vi "Popup.vi"(8 "error in (no error)":errorcluster, 10 "MSG":string, 11 "Popup in":refnum<class "Popup.lvclass">) -> (0 "error out":errorcluster, 3 "Popup out":refnum<class "Popup.lvclass">)   [LabVIEW 2020, in "Test-Client.lvlib" / "Popup.lvclass"]
uses:
  Popup.lvclass
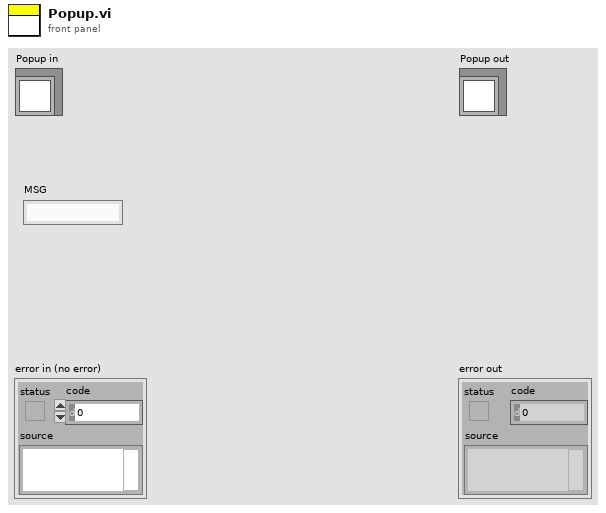
[diagram p1: front panel]
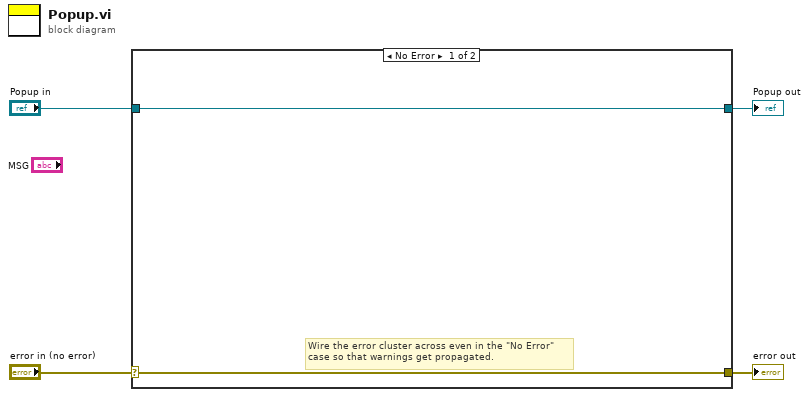
[diagram p0: block diagram]
diagram:
  n1 = case shown="No Error" "error in (no error)" {
    selector: "error in (no error)" -> [w5 w8]
    tunnel: [w5 w8] -> w3
    tunnel: [w6 w7] -> w1
    tunnel: "Popup in" -> [w6 w7]
    frame No Error {
      # "Wire the error cluster across even in the \"No Error\"\ncase so that warnings get propagated."
    }
    frame Error {
    }
  }
  "error out" <- w3
  "Popup out" <- w1
